vi "P_control.vi"(8 "Kp":dbl=150.0 format="%#_13g", 11 "Feedback error":dbl[](array[numeric])) -> (3 "P control":dbl[](array[numeric]))   [LabVIEW 2021, in "System.lvclass"]
uses:
  System.lvclass
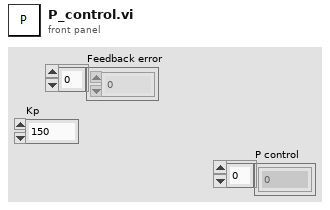
[diagram p1: front panel]
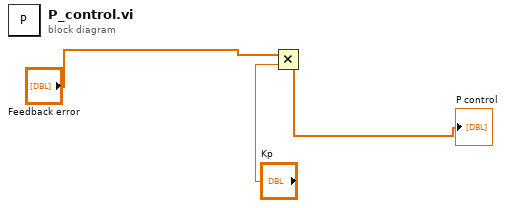
[diagram p0: block diagram]
diagram:
  n1 = Multiply(x="Feedback error", y="Kp") -> (x*y=→"P control":dbl[])
